vi "Configure EditPabel.vi"(8 "error in (no error)":errorcluster, 9 "Panel":refnum<class "Panel Controller Interface.lvclass">, 10 "vi reference":refnum<vi>) -> (0 "error out":errorcluster, 3 "EditPanel out":refnum<class "EditPanel API.lvclass">)   [LabVIEW 2015, in "EditPanel API.lvlib" / "EditPanel API.lvclass"]
uses:
  EditPanel API.lvclass
  Panel Control_Interface/Panel_interface/Panel Controller Interface.lvclass
  Console/Console.lvclass
  Console Reply/Console Reply/Console Reply.lvclass
  myPanel/Panel Control_Ref/Panel Controller.lvclass
  Console Reply/Console Reply/Console Reply.lvclass/Console Reply.ctl
  Console/Console.lvclass/Console.ctl
  EditPanel API.lvclass/EditPanel API.ctl
  <vilib>/ActorFramework/Actor/Actor.lvclass
  <vilib>/Utility/error.llb/Error Cluster From Error Code.vi
  <vilib>/ErrorRing/Error Ring.xnode
panel:
  out "x = y?":bool
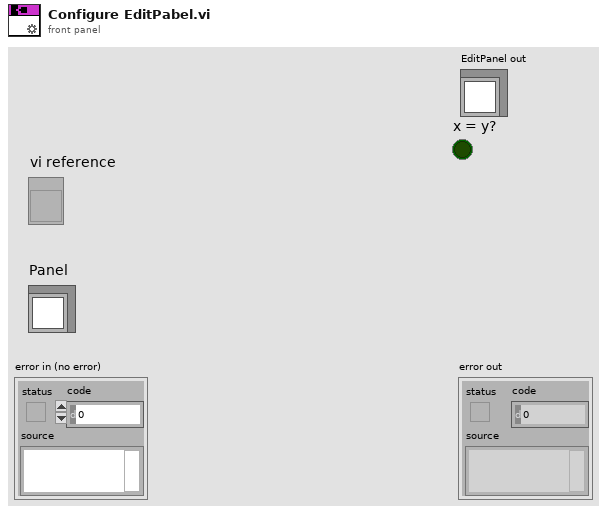
[diagram p1: front panel]
types:
  T1 = typedef "EditPanel API.lvlib/Console.lvclass/Console_Q Data Type.ctl" = cluster{"Console Reply":refnum<class "Console Reply.lvclass">, "Panel":refnum<class "Panel Controller Interface.lvclass">}
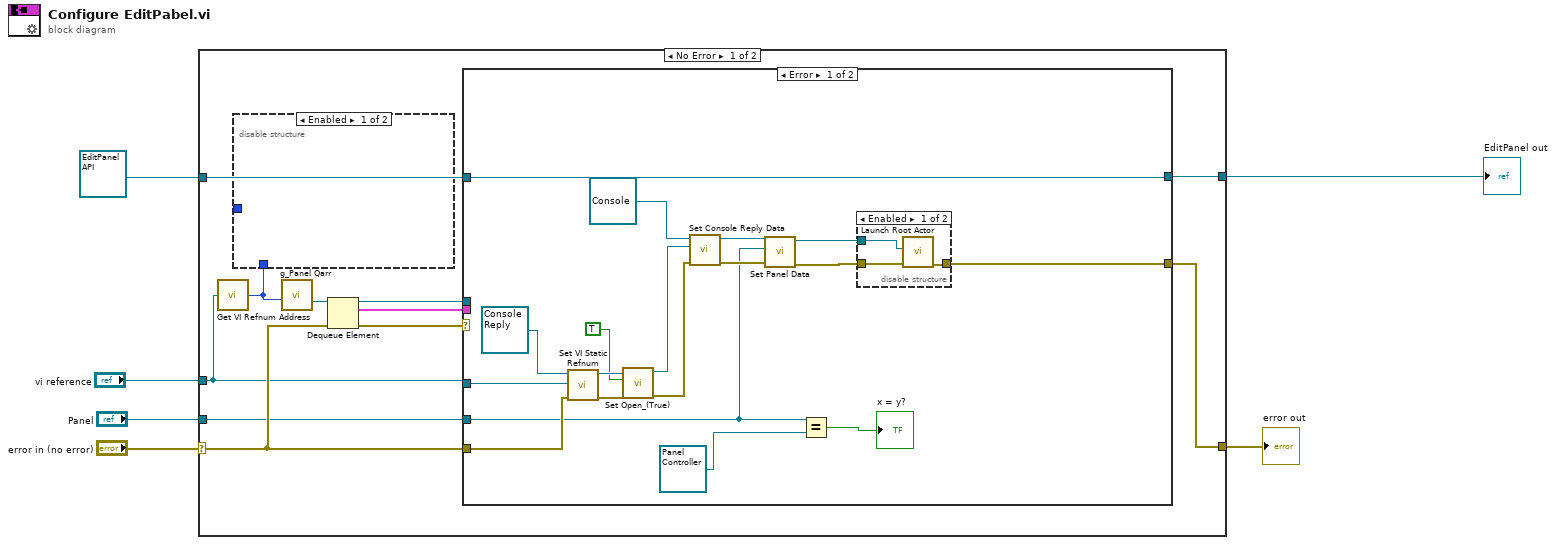
[diagram p0: block diagram]
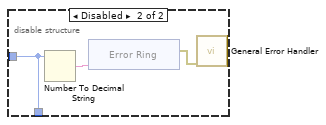
[diagram p2: hidden frame]
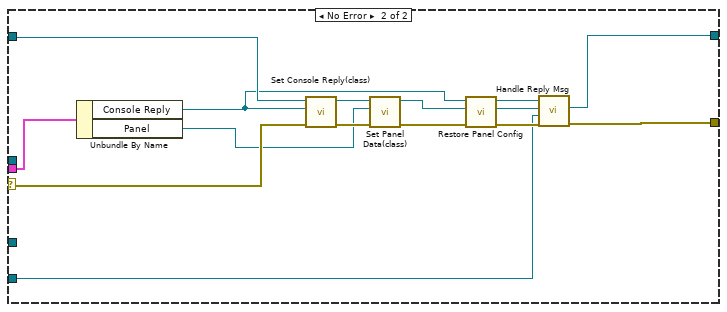
[diagram p4: hidden frame]
diagram:
  n1 = case shown="No Error" "error in (no error)" {
    selector: "error in (no error)" -> [w14 w66]
    tunnel: [w17 w65] -> w5
    tunnel: [w16 w66] -> w4
    tunnel: refnum<class "EditPanel API.lvclass"> refnum ("EditPanel in") -> [w15 w65]
    tunnel: "vi reference" -> [w10 _]
    tunnel: "Panel" -> [w7 _]
    frame No Error {
      n2 = call "Get VI Refnum Address.vi"("VI Refnum"=w10) -> ("Get Ref Address"=w8:u16)
      n3 = disable-structure shown="Enabled" {
        disable-tunnel: [_ w18] -> _
        disable-tunnel: w8 -> [_ w18]
        frame Enabled {
        }
        frame Disabled {
          n4 = Number To Decimal String(number=w18) -> (decimal integer string=w20:string)  [unwired: 1 in]
          n5 = xnode "Error Ring"("parameter 0"=w20) -> ("error out"=w19:errorcluster)
          n6 = call <vilib>:"General Error Handler.vi"("error in (no error)"=w19) -> ()  [unwired: 10 in, 5 out]
        }
      }
      n7 = call "g_Panel Qarr.vi"("VI Address"=w8) -> ("Console Q out"=w11:refnum<queue>)  [unwired: 10 in]
      n8 = Dequeue Element(queue=w11, error in (no error)=w14) -> (queue out=w13:refnum<queue>, element=w12:T1, error out=w9:errorcluster)  [unwired: 1 in, 1 out]
      n9 = case shown="Error" w9 {
        selector: w9 -> [_ w53]
        tunnel: w10 -> [w37 _]
        tunnel: w15 -> [w45 w62]
        tunnel: [w45 w64] -> w17
        tunnel: [w44 w52] -> w16
        tunnel: w14 -> [w36 _]
        tunnel: w13 -> [_ _]
        tunnel: w12 -> [_ w63]
        tunnel: w7 -> [w30 w50]
        frame Error {
          n10 = call "Set VI Static Refnum.vi"("error in (no error)"=w36, "VI Static Refnum"=w37, "Console Reply in"=refnum<class "Console Reply.lvclass"> refnum ("Console Reply.lvclass")) -> ("error out"=w34:errorcluster, "Console Reply out"=w35:refnum<class "Console Reply.lvclass">)  [unwired: 7 in]
          n11 = call "Set Open_(True).vi"("error in (no error)"=w34, "Open?(True)"=TRUE, "Console Reply in"=w35) -> ("error out"=w32:errorcluster, "Console Reply out"=w33:refnum<class "Console Reply.lvclass">)  [unwired: 7 in]
          n12 = call "Set Console Reply Data.vi"("error in (no error)"=w32, "Console Reply.lvclass"=w33, "Console in"=refnum<class "Console.lvclass"> refnum ("Console.lvclass")) -> ("error out"=w41:errorcluster, "Console out"=w42:refnum<class "Console.lvclass">)  [unwired: 7 in]
          n13 = call "Set Panel Data.vi"("error in (no error)"=w41, "Panel"=w30, "Console in"=w42) -> ("error out"=w40:errorcluster, "Console out"=w39:refnum<class "Console.lvclass">)  [unwired: 7 in]
          n14 = Equal?(x=w30, y=refnum<class "Panel Controller.lvclass"> refnum ("Panel Control_Ref")) -> (x = y?=→"x = y?":bool)
          n15 = disable-structure shown="Enabled" {
            disable-tunnel: [w47 w49] -> w44
            disable-tunnel: w39 -> [w48 _]
            disable-tunnel: w40 -> [w46 w49]
            frame Enabled {
              n16 = call <vilib>:"Launch Root Actor.vi"("error in (no error)"=w46, "Actor"=w48) -> ("error out"=w47:errorcluster)  [unwired: 8 in, 1 out]
            }
            frame Disabled {
            }
          }
        }
        frame No Error {
          n17 = Unbundle By Name(w63) -> ("Console Reply"=w54:refnum<class "Console Reply.lvclass">, "Panel"=w51:refnum<class "Panel Controller Interface.lvclass">)
          n18 = call "Set Console Reply(class).vi"("error in (no error)"=w53, "Console Reply.lvclass"=w54, "EditPanel API in"=w62) -> ("error out"=w60:errorcluster, "EditPanel API out"=w61:refnum<class "EditPanel API.lvclass">)  [unwired: 7 in]
          n19 = call "Set Panel Data(class).vi"("error in (no error)"=w60, "Panel"=w51, "EditPanel API in"=w61) -> ("error out"=w58:errorcluster, "EditPanel API out"=w59:refnum<class "EditPanel API.lvclass">)  [unwired: 7 in]
          n20 = call "Restore Panel Config.vi"("error in (no error)"=w58, "EditPanel API in"=w59, "Console Reply in"=w54) -> ("error out"=w55:errorcluster, "EditPanel API out"=w56:refnum<class "EditPanel API.lvclass">, "Console Reply out"=w57:refnum<class "Console Reply.lvclass">)  [unwired: 6 in]
          n21 = call-dynamic "Handle Reply Msg.vi"("error in (no error)"=w55, "Panel Controller"=w50, "EditPanel API in"=w56, "Console Reply"=w57) -> ("error out"=w52:errorcluster, "EditPanel API out"=w64:refnum<class "EditPanel API.lvclass">)  [unwired: 6 in]
        }
      }
    }
    frame Error {
    }
  }
  "error out" <- w4
  "EditPanel out" <- w5
